vi "Get System Metrics.vi"(8 "error in (no error)":errorcluster) -> (0 "error out":errorcluster, 2 "Y":i32, 3 "X":i32)   [LabVIEW 2019]
uses:
  user32.dll
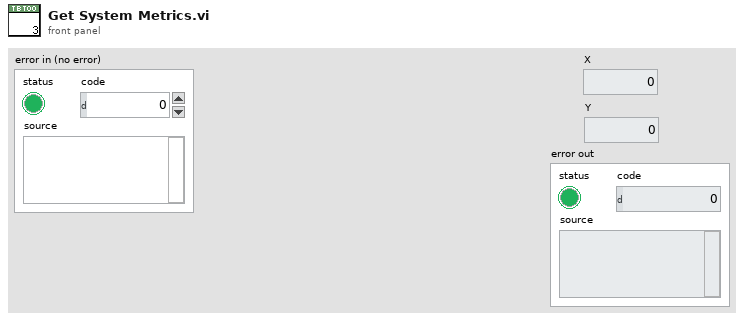
[diagram p1: front panel]
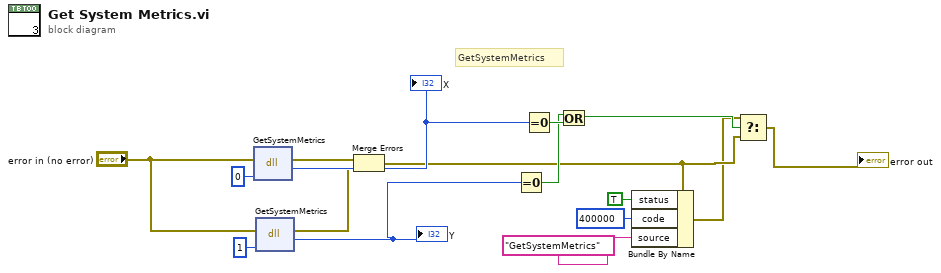
[diagram p0: block diagram]
diagram:
  # "GetSystemMetrics"
  n1 = dll-call lib="user32.dll" fn="GetSystemMetrics"(error in="error in (no error)", "nIndex"=0) -> (error out=w9:errorcluster, "return"=w16:i32)  [unwired: 3 in, 1 out]
  "X" <- w16
  n2 = dll-call lib="user32.dll" fn="GetSystemMetrics"(error in="error in (no error)", "nIndex"=1) -> (error out=w8:errorcluster, "return"=w11:i32)  [unwired: 3 in, 1 out]
  "Y" <- w11
  n3 = Merge Errors(w9, w8) -> (w2:errorcluster)
  n4 = Equal To 0?(x=w11) -> (x = 0?=w10:bool)
  n5 = Equal To 0?(x=w16) -> (x = 0?=w15:bool)
  n6 = Or(x=w10, y=w15) -> (x .or. y?=w5:bool)
  n7 = Bundle By Name(cluster=w2, "status"=TRUE, "code"=400000, "source"="GetSystemMetrics") -> (w1:errorcluster)
  n8 = Select(t=w1, s=w5, f=w2) -> (s? t:f=→"error out":errorcluster)
